vi "5900PRSet.vi"(11 "ExitSendCmd":bool) -> (4 "Panametrics Settings Out":T1={"ENERGY (uJ)"=0, "DAMPING (Ohm)"=0, "HP FILT (KHz) "=0, "LP FILT (MHz)"=0, "MODE"=0, "PRF (KHz)"=1, "GAIN (db)"=0, "COARSE ATTENUATION"=0, "FINE ATTENUATION"=0} {"FINE ATTENUATION" items=["00.0", "00.5", "01.0", "01.5", "02.0", "02.5", "03.0", "03.5", "04.0", "04.5", "05.0", "05.5", "06.0", "06.5", "07.0", "07.5", "08.0", "08.5", "09.0", "09.5", "10.0", "10.5", "11.0", "11.5", "12.0", "12.5", "13.0", "13.5", "14.0", "14.5", "15.0", "15.5"]; "COARSE ATTENUATION" items=["00.0", "10.0", "20.0", "30.0", "40.0", "50.0"]; "GAIN (db)" items=["26.0", "40.0", "54.0"]; "PRF (KHz)" items=["XREMT", "EXBNC", "0.200", "0.500", "1.000", "2.000", "5.000", "10.00", "20.00"]; "MODE" items=["P/ E", "THRU", "RPP", "EXT_PLSR"]; "LP FILT (MHz)" items=["20", "50", "100", "200"]; "HP FILT (KHz)" items=["1", "1000", "3000", "10000"]; "DAMPING (Ohm)" items=["7", "10", "16", "20", "26", "30", "40", "50"]; "ENERGY (uJ)" items=["1", "2", "4", "8", "16", "32"]}, 10 "Panametrics Address":refnum<visa-resource-name>="GPIB1::1::INSTR", 15 "no 5900?":bool)   [LabVIEW 2022 SP3]
doc: "This application VI allows the user to set the desired parameters in the \n5800 / 5900 P / R. just select thevalues that you want to set the instrument to from the 5800 / 5900 user interface and click on the send to 5800 button."
uses:
  Pana5900.ctl
  PulserGlobals.vi
panel:
  in  "Panametrics Settings":T1={"ENERGY (uJ)"=0, "DAMPING (Ohm)"=0, "HP FILT (KHz) "=0, "LP FILT (MHz)"=0, "MODE"=0, "PRF (KHz)"=1, "GAIN (db)"=0, "COARSE ATTENUATION"=0, "FINE ATTENUATION"=0} {"FINE ATTENUATION" items=["00.0", "00.5", "01.0", "01.5", "02.0", "02.5", "03.0", "03.5", "04.0", "04.5", "05.0", "05.5", "06.0", "06.5", "07.0", "07.5", "08.0", "08.5", "09.0", "09.5", "10.0", "10.5", "11.0", "11.5", "12.0", "12.5", "13.0", "13.5", "14.0", "14.5", "15.0", "15.5"]; "COARSE ATTENUATION" items=["00.0", "10.0", "20.0", "30.0", "40.0", "50.0"]; "GAIN (db)" items=["26.0", "40.0", "54.0"]; "PRF (KHz)" items=["XREMT", "EXBNC", "0.200", "0.500", "1.000", "2.000", "5.000", "10.00", "20.00"]; "MODE" items=["P/ E", "THRU", "RPP", "EXT_PLSR"]; "LP FILT (MHz)" items=["20", "50", "100", "200"]; "HP FILT (KHz)" items=["1", "1000", "3000", "10000"]; "DAMPING (Ohm)" items=["7", "10", "16", "20", "26", "30", "40", "50"]; "ENERGY (uJ)" items=["1", "2", "4", "8", "16", "32"]}
  out "ATTENUATORS(db)":dbl format="%.2f"
  # "MODEL 5900"
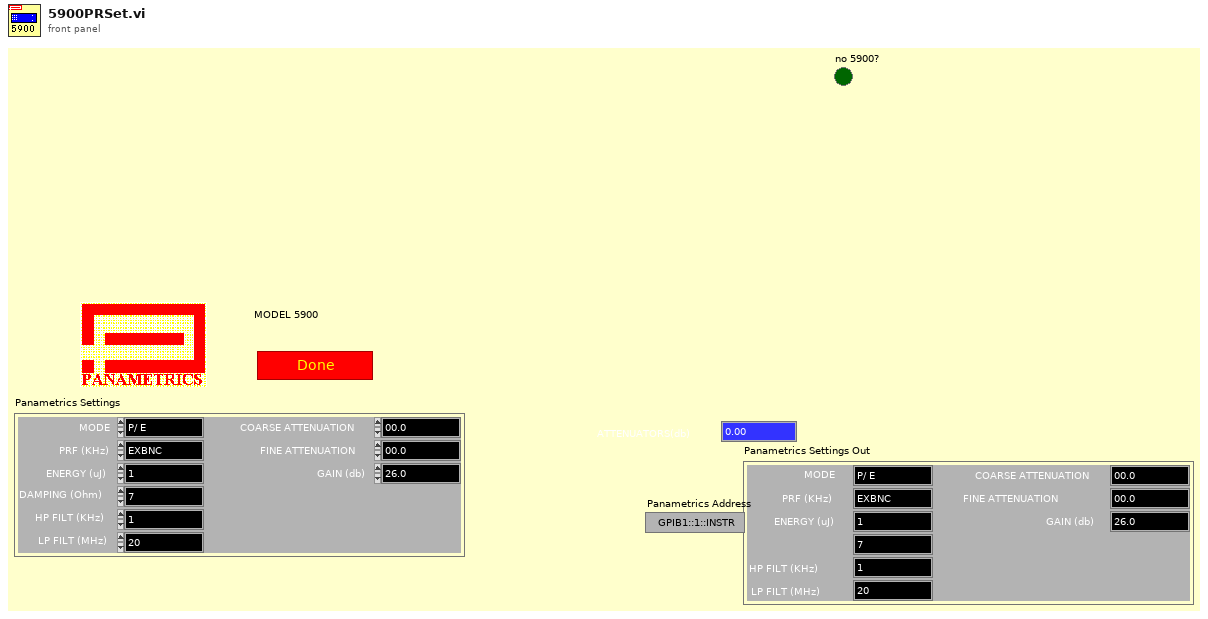
[diagram p1: front panel]
types:
  T1 = typedef "Pana5900.ctl" = cluster{"ENERGY (uJ)":u16, "DAMPING (Ohm)":u16, "HP FILT (KHz) ":u16, "LP FILT (MHz)":u16, "MODE":u16, "PRF (KHz)":u16, "GAIN (db)":u16, "COARSE ATTENUATION":u16, "FINE ATTENUATION":u16}
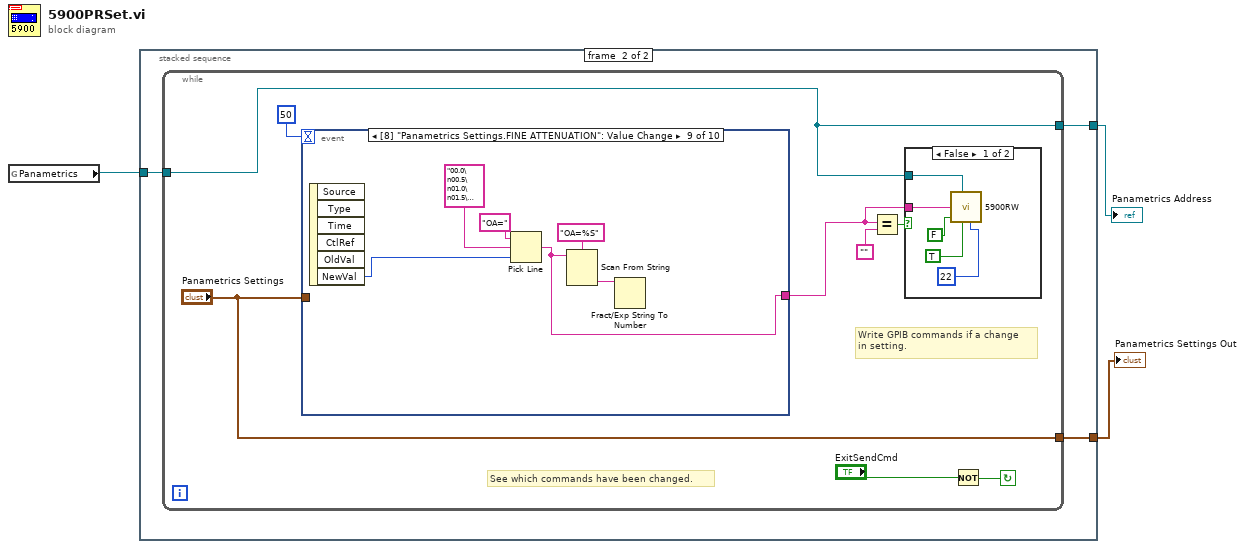
[diagram p0: block diagram]
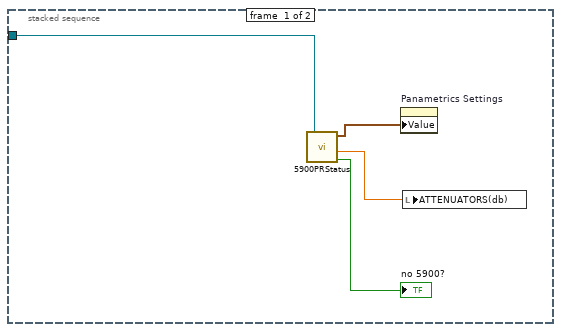
[diagram p2: hidden frame]
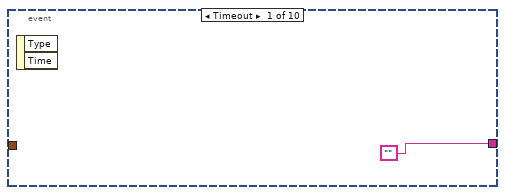
[diagram p4: hidden frame]
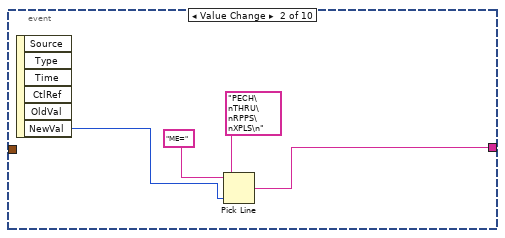
[diagram p5: hidden frame]
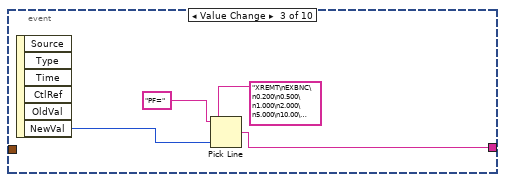
[diagram p6: hidden frame]
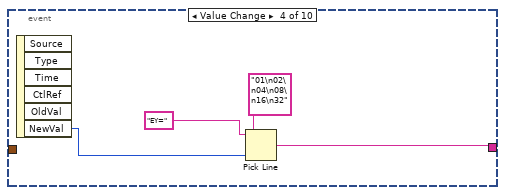
[diagram p7: hidden frame]
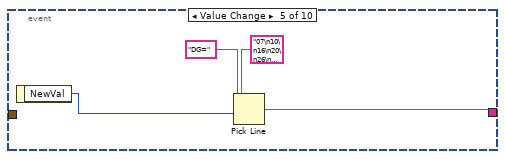
[diagram p8: hidden frame]
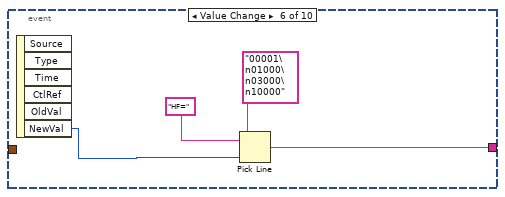
[diagram p9: hidden frame]
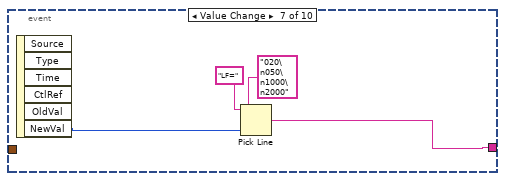
[diagram p10: hidden frame]
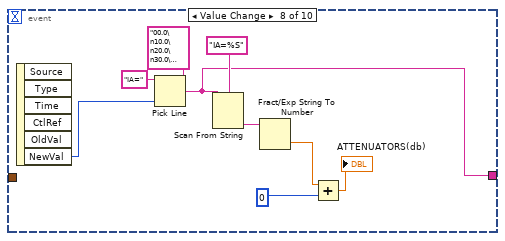
[diagram p11: hidden frame]
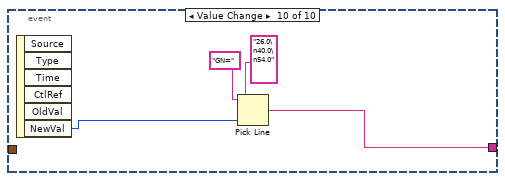
[diagram p12: hidden frame]
diagram:
  n1 = global read "PulserGlobals.vi" "Panametrics"() -> (w1:refnum<visa-resource-name>)
  n2 = stacked-sequence {
    tunnel: w1 -> [w7 w10]
    tunnel: [_ w9] -> w3
    tunnel: [_ w8] -> w2
    frame #0 {
      n3 = call "5900PRStatus.vi"("VISA resource name"=w7) -> ("Panametrics Settings"=w4:T1, "ATTENUATORS(db)"=w6:dbl, "no 5900?"=→"no 5900?":bool)  [unwired: 1 in, 1 out]
      n4 = property on="Panametrics Settings" class="Clust (strict)"("Value"=w4) -> ()  [unwired: 2 in, 2 out]
      n5 = local write "ATTENUATORS(db)"(w6) -> ()
    }
    frame #1 {
      n6 = while {
        tunnel: w10 -> [w11]
        tunnel: ["Panametrics Settings"] -> w9
        tunnel: [w11] -> w8
        stop <- w18 continue-if-true
        # "Write GPIB commands if a change\nin setting."
        # "See which commands have been changed."
        n7 = event shown="[8] \"Panametrics Settings.FINE ATTENUATION\": Value Change" {
          selector: _ -> [_ _ _ _ _ _ _ _ _ _]
          dyn-events: _ -> [_ _ _ _ _ _ _ _ _ _]
          timeout: 50 -> [_ _ _ _ _ _ _ _ _ _]
          tunnel: ["" w26 w30 w34 w38 w42 w46 w51 w59 w65] -> w15
          tunnel: "Panametrics Settings" -> [_ _ _ _ _ _ _ _ _ _]
          event Timeout {
            n8 = event-data() -> ()  [unwired: 3 out]
          }
          event Value Change {
            n9 = event-data() -> ("NewVal"=w25:u16)  [unwired: 6 out]
            n10 = Pick Line(string ("")="ME=", multi-line string="PECH\nTHRU\nRPPS\nXPLS\n", line index=w25) -> (output string=w26:string)
          }
          event Value Change {
            n11 = event-data() -> ("NewVal"=w29:u16)  [unwired: 6 out]
            n12 = Pick Line(string ("")="PF=", multi-line string="XREMT\nEXBNC\n0.200\n0.500\n1.000\n2.000\n5.000\n10.00\n20.00\n", line index=w29) -> (output string=w30:string)
          }
          event Value Change {
            n13 = event-data() -> ("NewVal"=w33:u16)  [unwired: 6 out]
            n14 = Pick Line(string ("")="EY=", multi-line string="01\n02\n04\n08\n16\n32", line index=w33) -> (output string=w34:string)
          }
          event Value Change {
            n15 = event-data() -> ("NewVal"=w37:u16)  [unwired: 1 out]
            n16 = Pick Line(string ("")="DG=", multi-line string="07\n10\n16\n20\n26\n30\n40\n50\n", line index=w37) -> (output string=w38:string)
          }
          event Value Change {
            n17 = event-data() -> ("NewVal"=w41:u16)  [unwired: 6 out]
            n18 = Pick Line(string ("")="HF=", multi-line string="00001\n01000\n03000\n10000", line index=w41) -> (output string=w42:string)
          }
          event Value Change {
            n19 = event-data() -> ("NewVal"=w45:u16)  [unwired: 6 out]
            n20 = Pick Line(string ("")="LF=", multi-line string="020\n050\n1000\n2000", line index=w45) -> (output string=w46:string)
          }
          event Value Change {
            n21 = event-data() -> ("NewVal"=w49:u16)  [unwired: 6 out]
            n22 = Pick Line(string ("")="IA=", multi-line string="00.0\n10.0\n20.0\n30.0\n40.0\n50.0\n60.0", line index=w49) -> (output string=w51:string)
            n23 = Scan From String(format string="IA=%S", input string=w51) -> (output 1=w52:string)  [unwired: 2 in, 4 out]
            n24 = Fract/Exp String To Number(string=w52) -> (number=w56:dbl)  [unwired: 4 out]
            n25 = Add(x=w56, y=0) -> (x+y=→"ATTENUATORS(db)":dbl)
          }
          event Value Change {
            n26 = event-data() -> ("NewVal"=w58:u16)  [unwired: 6 out]
            n27 = Pick Line(string ("")="OA=", multi-line string="00.0\n00.5\n01.0\n01.5\n02.0\n02.5\n03.0\n03.5\n04.0\n04.5\n05.0\n05.5\n06.0\n06.5\n07.0\n07.5\n08.0\n08.5\n09.0\n09.5\n10.0\n10.5\n11.0\n11.5\n12.0\n12.5\n13.0\n13.5\n14.0\n14.5\n15.0\n15.5", line index=w58) -> (output string=w59:string)
            n28 = Scan From String(format string="OA=%S", input string=w59) -> (output 1=w60:string)  [unwired: 2 in, 4 out]
            n29 = Fract/Exp String To Number(string=w60) -> ()  [unwired: 5 out]
          }
          event Value Change {
            n30 = event-data() -> ("NewVal"=w64:u16)  [unwired: 6 out]
            n31 = Pick Line(string ("")="GN=", multi-line string="26.0\n40.0\n54.0", line index=w64) -> (output string=w65:string)
          }
        }
        n32 = Equal?(x=w15, y="") -> (x = y?=w14:bool)
        n33 = case shown="False" w14 {
          tunnel: w15 -> [w23 _]
          tunnel: w11 -> [w20 _]
          frame False {
            n34 = call "5900RW.vi"("VISA resource name"=w20, "ENTER STRING"=w23, "Read ?"=FALSE, "Write ?"=TRUE, "# bytes\nto read"=22) -> ()  [unwired: 5 out]
          }
          frame True {
          }
        }
        n35 = Not(x="ExitSendCmd") -> (.not. x?=w18:bool)
      }
    }
  }
  "Panametrics Settings Out" <- w3
  "Panametrics Address" <- w2
